vi "Get Version.vi"(8 "error in (no error)":errorcluster, 11 "system in":refnum<class "Systems.lvclass">) -> (0 "error out":errorcluster, 2 "version":T1, 3 "system out":refnum<class "Systems.lvclass">)   [LabVIEW 2013, in "PL Framework Configuration Tool.lvlib" / "Systems.lvclass"]
uses:
  Systems.lvclass
  Systems.lvclass/Systems.ctl
  Framework Configuration Classes/system configuration/PL_System Configuration.lvclass/PL_System Configuration.ctl
  Framework Configuration Classes/system configuration/PL_System Configuration.lvclass
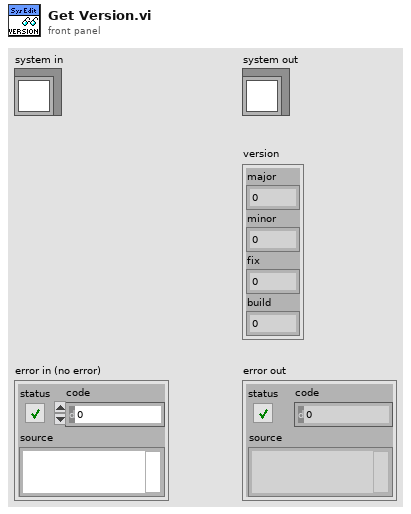
[diagram p1: front panel]
types:
  T1 = cluster{"major":u16, "minor":u16, "fix":u16, "build":u16}
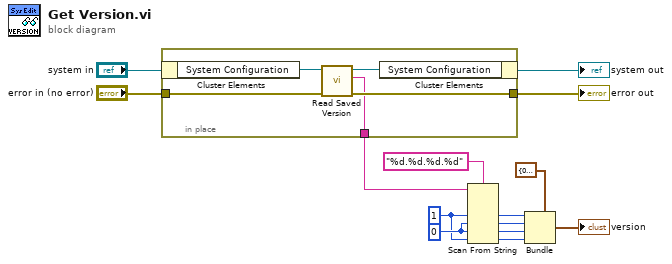
[diagram p0: block diagram]
diagram:
  w9 = u16 0
  w8 = u16 1
  n1 = in-place {
    in-place-border: "error in (no error)" -> [w19]
    in-place-border: [w18] -> w11
    in-place-border: [w15] -> w7
    n2 = in-place-cluster #1("system in") -> ("System Configuration"=w17:refnum<class "PL_System Configuration.lvclass">)
    n3 = call "Read Saved Version.vi"("error in"=w19, "PL_System Configuration in"=w17) -> ("error out"=w18:errorcluster, "Saved Version"=w15:string, "PL_System Configuration out"=w16:refnum<class "PL_System Configuration.lvclass">)  [unwired: 7 in]
    n4 = in-place-cluster #1("System Configuration"=w16) -> (→"system out":refnum<class "Systems.lvclass">)
  }
  "error out" <- w11
  n5 = Scan From String(format string="%d.%d.%d.%d", input string=w7, default 1=w8, default 2=w9, default 3=w9, default 4=w8) -> (output 1=w5:u16, output 2=w4:u16, output 3=w3:u16, output 4=w2:u16)  [unwired: 2 in, 3 out]
  n6 = Bundle(cluster=T1 {"major"=0, "minor"=0, "fix"=0, "build"=0} ("version"), "major"=w5, "minor"=w4, "fix"=w3, "build"=w2) -> (→"version":T1)
